vi "Read ImData.vi"(8 "error in (no error)":errorcluster, 10 "ReadSize":u32, 11 "AODAcq in":refnum<class "AODAcq.lvclass">) -> (0 "error out":errorcluster, 2 "ImData":waveform(i32)[](array[waveform]), 3 "AODAcq out":refnum<class "AODAcq.lvclass">)   [LabVIEW 2014, in "AODAcq.lvclass"]
uses:
  AODAcq.lvclass
  AODAcq.lvclass/AODAcq.ctl
  <vilib>/Utility/error.llb/Error Cluster From Error Code.vi
  <vilib>/rvi/errors/niLvFpgaAdjustHostInterfaceError.vi
  HDF5Tools/LabView/Append To Dataset 2D Double.vi
  <vilib>/rvi/interface/nirviMethod/nirviMethod.xnode
  FPGA_Control/AODRef.ctl
  FPGA Bitfiles/AodScanner_FPGATarget_AODControl(FPGA)_TyJc9yYmyGA.lvbitx
  HDF5Tools/LabView/HDF5Tools.lvlib
  <vilib>/rvi/errors/niLvFpgaMergeErrorWithErrorCode.vi
  <vilib>/FPGAPlugInAG/PXIe-7965R/niLvFpga_ReadFifo_PXIe-7965R.vi
panel:
  out "Samples":i32
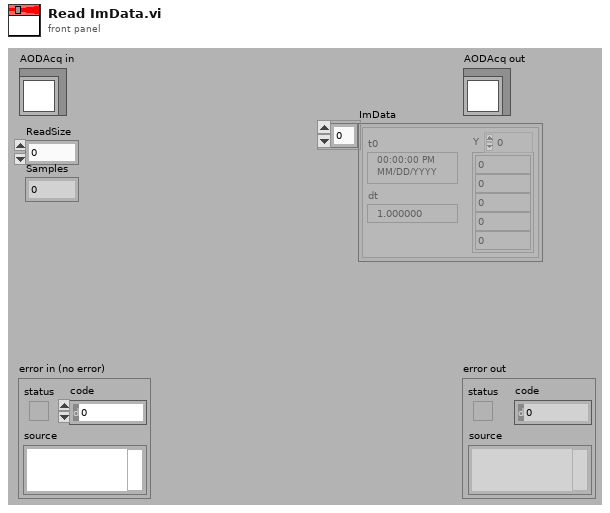
[diagram p1: front panel]
types:
  T1 = typedef "AODRef.ctl" = refnum<k20>
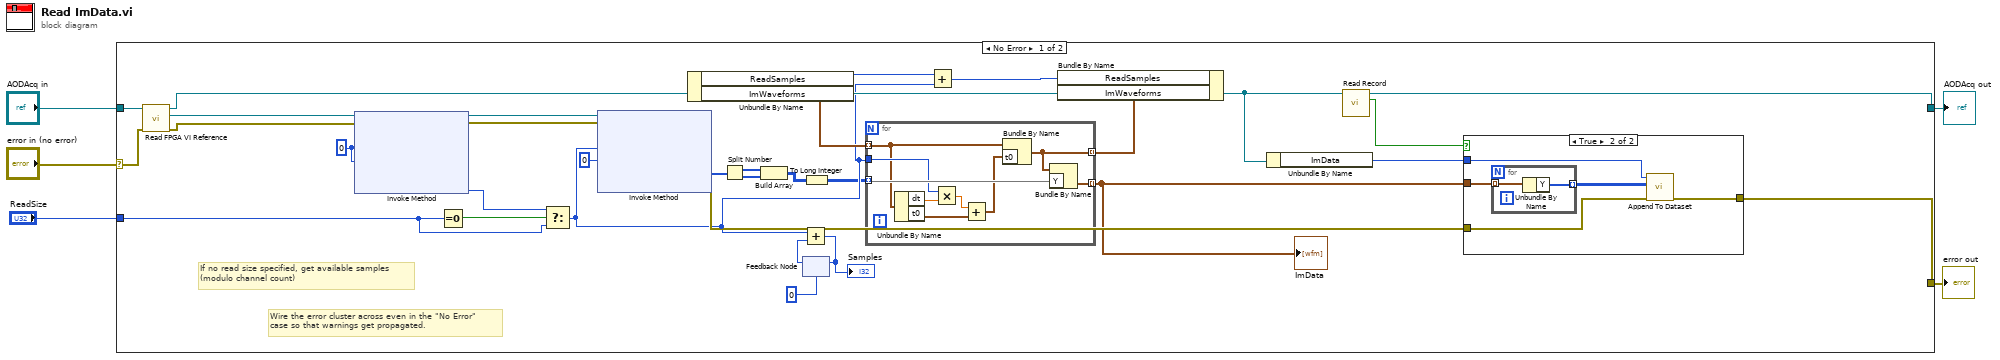
[diagram p0: block diagram]
diagram:
  n1 = case shown="No Error" "error in (no error)" {
    selector: "error in (no error)" -> [w31 w56]
    tunnel: [w25 w56] -> w4
    tunnel: [w8 w55] -> w2
    tunnel: "AODAcq in" -> [w37 w55]
    tunnel: "ReadSize" -> [w19 _]
    frame No Error {
      w36 = u32 0 ("Number of Elements")
      # "If no read size specified, get available samples \n(modulo channel count)"
      # "Wire the error cluster across even in the \"No Error\"\ncase so that warnings get propagated."
      n2 = call-dynamic "Read FPGA VI Reference.vi"("error in (no error)"=w31, "AODAcq in"=w37) -> ("error out"=w12:errorcluster, "FPGA VI Reference"=w13:T1, "AODAcq out"=w29:refnum<class "AODAcq.lvclass">)  [unwired: 7 in]
      n3 = xnode "Invoke Method"("FPGA VI Reference In"=w13, "error in"=w12, "Number of Elements"=w36, "Timeout (ms)"=w36) -> ("FPGA VI Reference Out"=w34:T1, "error out"=w33:errorcluster, "Elements Remaining"=w15:u32)  [unwired: 1 out]
      n4 = Equal To 0?(x=w19) -> (x = 0?=w35:bool)
      n5 = Select(t=w15, s=w35, f=w19) -> (s? t:f=w16:u32)
      n6 = xnode "Invoke Method"("FPGA VI Reference In"=w34, "error in"=w33, "Number of Elements"=w16, "Timeout (ms)"=0) -> ("error out"=w26:errorcluster, "Data"=w18:u64[])  [unwired: 2 out]
      n7 = Unbundle By Name(w29) -> ("ReadSamples"=w24:u64, "ImWaveforms"=w30:waveform(i32)[])
      n8 = Split Number(x=w18) -> (hi(x)=w11:u32[], lo(x)=w10:u32[])
      n9 = Build Array(w11, w10) -> (w17:u32[][])
      n10 = feedback #1(0) -> (w21:i32)
      n11 = Add(x=w16, y=w21) -> (x+y=w22:u32)
      "Samples" <- w22
      n12 = feedback-in #1(w22) -> ()
      n13 = To Long Integer(number=w17) -> (32bit integer=w14:i32[][])
      n14 = for {
        tunnel: w14 -> [w54] mode=indexing
        tunnel: [w53] -> w6 mode=indexing
        tunnel: w30 -> [w48] mode=indexing
        tunnel: w16 -> [w51]
        tunnel: [w46] -> w28 mode=indexing
        n15 = Unbundle By Name(w48) -> ("dt"=w52:dbl, "t0"=w49:timestamp)
        n16 = Multiply(x=w51, y=w52) -> (x*y=w50:dbl)
        n17 = Add(x=w50, y=w49) -> (x+y=w47:timestamp)
        n18 = Bundle By Name(cluster=w48, "t0"=w47) -> (w46:waveform(i32))
        n19 = Bundle By Name(cluster=w46, "Y"=w54) -> (w53:waveform(i32))
      }
      "ImData" <- w6
      n20 = Add(x=w24, y=w16) -> (x+y=w23:u64)
      n21 = Bundle By Name(cluster=w29, "ReadSamples"=w23, "ImWaveforms"=w28) -> (w9:refnum<class "AODAcq.lvclass">)
      n22 = Unbundle By Name(w9) -> ("ImData"=w27:i32)
      n23 = call-dynamic "Read Record.vi"("AODAcq in"=w9) -> ("Record"=w7:bool, "AODAcq out"=w8:refnum<class "AODAcq.lvclass">)  [unwired: 8 in, 1 out]
      n24 = case shown="True" w7 {
        tunnel: w6 -> [_ w43]
        tunnel: w27 -> [_ w40]
        tunnel: w26 -> [w38 w41]
        tunnel: [w38 w39] -> w25
        frame False {
        }
        frame True {
          n25 = for {
            tunnel: w43 -> [w45] mode=indexing
            tunnel: [w44] -> w42 mode=indexing
            n26 = Unbundle By Name(w45) -> ("Y"=w44:i32[])
          }
          n27 = call-poly "Append To Dataset.vi"("Error in (no error)"=w41, "Data"=w42, "Dataset id in"=w40) -> ("Error out"=w39:errorcluster)  [unwired: 7 in, 1 out]
        }
      }
    }
    frame Error {
    }
  }
  "error out" <- w4
  "AODAcq out" <- w2
